vi "resetSelection.vi"(8 "error in (no error)":errorcluster, 10 "Selection":i32=-1, 11 "SingleSelectMCLBAdapter in":refnum<class "SingleSelectMCLBAdapter.lvclass">) -> (0 "error out":errorcluster, 3 "SingleSelectMCLBAdapter out":refnum<class "SingleSelectMCLBAdapter.lvclass">)   [LabVIEW 2020, in "SingleSelectMCLBAdapter.lvclass"]
uses:
  SingleSelectMCLBAdapter.lvclass
  SingleSelectMCLBAdapter.lvclass/SingleSelectMCLBAdapter.ctl
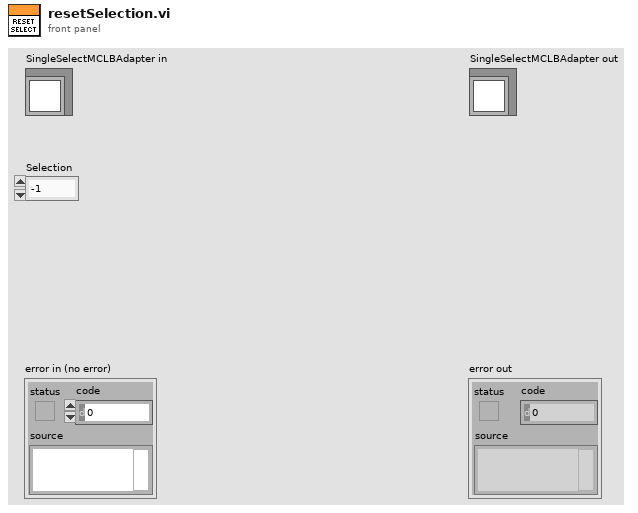
[diagram p1: front panel]
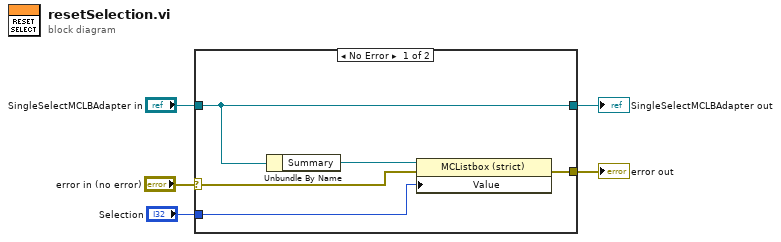
[diagram p0: block diagram]
diagram:
  n1 = case shown="No Error" "error in (no error)" {
    selector: "error in (no error)" -> [w7 w11]
    tunnel: [w8 w12] -> w4
    tunnel: [w10 w11] -> w3
    tunnel: "SingleSelectMCLBAdapter in" -> [w8 w12]
    tunnel: "Selection" -> [w6 _]
    frame No Error {
      n2 = Unbundle By Name(w8) -> ("Summary"=w9:refnum<vi>)
      n3 = property class="MCListbox (strict)"(reference=w9, error in=w7, "Value"=w6) -> (error out=w10:errorcluster)  [unwired: 1 out]
    }
    frame Error {
    }
  }
  "error out" <- w3
  "SingleSelectMCLBAdapter out" <- w4
